vi "Read Proceeding Dir.vi"(8 "error in (no error)":errorcluster, 11 "HIJ Vision File Viewer App in":refnum<class "HIJ Vision File Viewer App.lvclass">) -> (0 "error out":errorcluster, 2 "Proceeding Dir":bool, 3 "HIJ Vision File Viewer App out":refnum<class "HIJ Vision File Viewer App.lvclass">)   [LabVIEW 2014, in "HIJ Vision File Viewer App.lvlib" / "HIJ Vision File Viewer App.lvclass"]
uses:
  HIJ Vision File Viewer App.lvclass
  HIJ Vision File Viewer App.lvclass/HIJ Vision File Viewer App.ctl
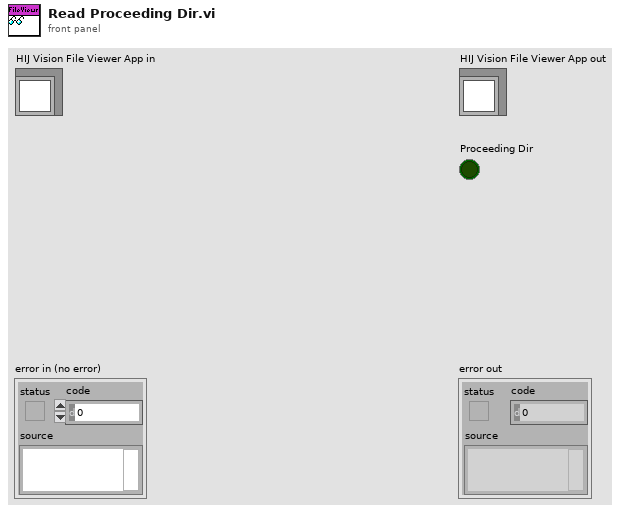
[diagram p1: front panel]
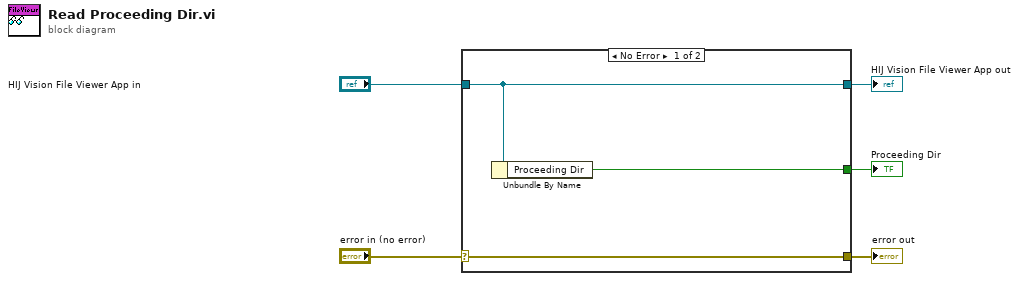
[diagram p0: block diagram]
diagram:
  n1 = case shown="No Error" "error in (no error)" {
    selector: "error in (no error)" -> [w8 w9]
    tunnel: [w8 w9] -> w4
    tunnel: [w7 w10] -> w2
    tunnel: "HIJ Vision File Viewer App in" -> [w7 w10]
    tunnel: [w6 _] -> w1
    frame No Error {
      n2 = Unbundle By Name(w7) -> ("Proceeding Dir"=w6:bool)
    }
    frame Error {
    }
  }
  "error out" <- w4
  "HIJ Vision File Viewer App out" <- w2
  "Proceeding Dir" <- w1
